vi "FarFiledPreCap.vi"(2 "error in (no error)":errorcluster caption="error in（no error）") -> (0 "error out":errorcluster)   [LabVIEW 2018]
panel:
  # "开始远场图像采集，预先采集五张"
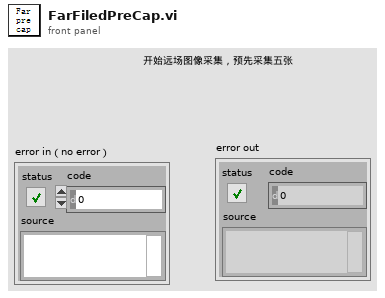
[diagram p1: front panel]
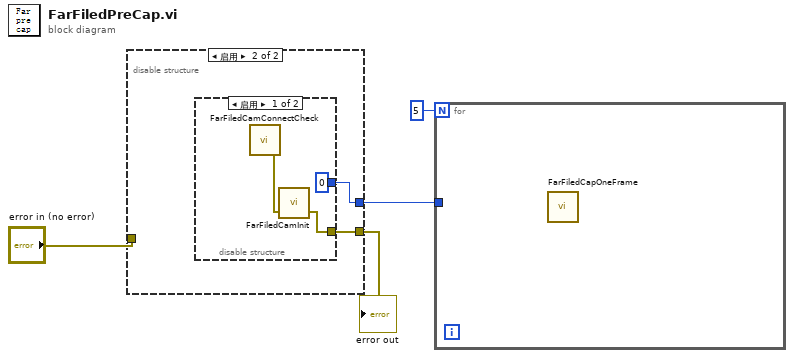
[diagram p0: block diagram]
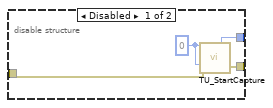
[diagram p2: hidden frame]
diagram:
  n1 = disable-structure shown="启用" {
    disable-tunnel: "error in (no error)" -> [w7 _]
    disable-tunnel: [w6 w10] -> w2
    disable-tunnel: [w5 w9] -> w1
    frame Disabled {
      w8 = u8 0 ("Camera Index")
      n2 = call "TU_StartCapture.vi"("Camera Index"=w8, "Capture Mode"=w8, "error in (no error)"=w7) -> ("ImageType"=w6:u32, "error out"=w5:errorcluster)  [unwired: 6 in, 5 out]
    }
    frame Enabled {
      n3 = disable-structure shown="启用" {
        disable-tunnel: [0 _] -> w10
        disable-tunnel: [w11 _] -> w9
        frame Enabled {
          n4 = call "FarFiledCamConnectCheck.vi"() -> ("error out"=w12:errorcluster)  [unwired: 2 in, 1 out]
          n5 = call "FarFiledCamInit.vi"("error in (no error)"=w12) -> ("error out"=w11:errorcluster)  [unwired: 2 in]
        }
        frame Disabled {
        }
      }
    }
  }
  "error out" <- w1
  n6 = for {
    N: 5 -> [_]
    tunnel: w2 -> [_]
    n7 = call "FarFiledCapOneFrame.vi"() -> ()  [unwired: 11 in, 1 out]
  }
